vi "main.vi"() -> ()   [LabVIEW 2025]
panel:
  out "pNN50":dbl
  out "NN50":i16
  out "RMSSD":dbl
  out "stdRR":dbl format="%0.2f"
  out "meanRR":dbl format="%0.5f"
  out "deltaTime":dbl[](array[numeric])
  out "Time":dbl[](array[numeric])
  out "HRV(t)":cluster{dbl[], dbl[]}(graph)
  out "deltaPeakTimes":dbl[](array[numeric])
  out "peakTimes":dbl[](array[numeric])
  out "2Dsignal/peaks":dbl[][](array[numeric])
  out "ECG w peaks":dynamicdata(graph)
  out "# peaks":dbl
  out "Raw ECG":dbl[](graph)
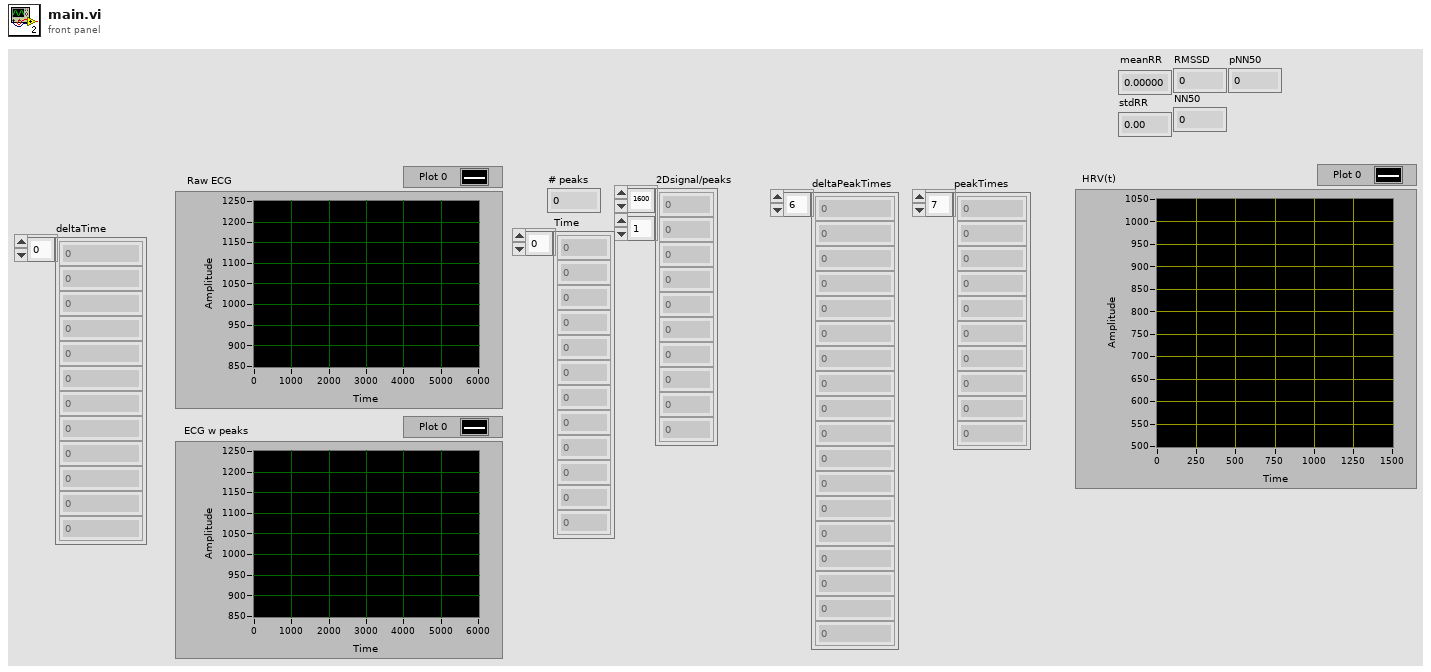
[diagram p1: front panel]
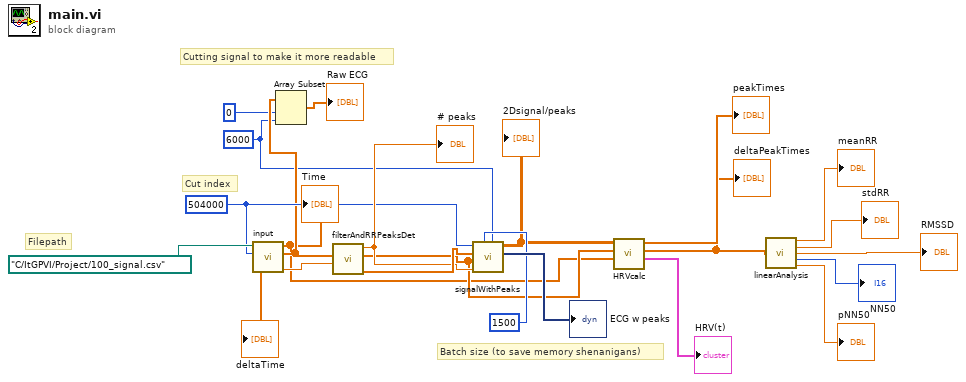
[diagram p0: block diagram]
diagram:
  w13 = 6000 ("length")
  w19 = 504000
  # "Batch size (to save memory shenanigans)"
  # "Cutting signal to make it more readable"
  # "Cut index"
  # "Filepath"
  n1 = call "input.vi"("cutIndex"=w19, "file path"=path "C:/ItGPVI/Project/100_signal.csv") -> ("fs"=w22:dbl, "ECG 1"=w16:dbl[], "Time"=w10:dbl[], "deltaTime"=→"deltaTime":dbl[])  [unwired: 4 in, 2 out]
  "Time" <- w10
  n2 = Array Subset(array=w16, index=0, length=w13) -> (→"Raw ECG":dbl[])
  n3 = call "filterAndRRPeaksDet.vi"("fs"=w22, "ECG1"=w16) -> ("Filtered ECG1"=w21:dbl[], "Locations"=w11:dbl[], "# peaks"=w20:dbl)  [unwired: 5 in, 2 out]
  "# peaks" <- w20
  n4 = call "signalWithPeaks.vi"("cutIndex"=w19, "filteredECG"=w21, "Locations"=w11, "# peaks"=w20, "batchSize"=1500, "lengthOfGraph"=w13) -> ("2Dsignal/peaks"=w12:dbl[][], "Waveform Graph"=→"ECG w peaks":dynamicdata)  [unwired: 3 in]
  "2Dsignal/peaks" <- w12
  n5 = call "HRVcalc.vi"("Time"=w10, "Locations"=w11, "2D"=w12) -> ("XY Graph"=→"HRV(t)":cluster{dbl[], dbl[]}, "deltaPeakTimes"=w6:dbl[], "peakTimes"=→"peakTimes":dbl[])  [unwired: 6 in]
  "deltaPeakTimes" <- w6
  n6 = call "linearAnalysis.vi"("deltaPeakTimes"=w6) -> ("meanRR"=→"meanRR":dbl, "stdRR"=→"stdRR":dbl, "RMSSD"=→"RMSSD":dbl, "NN50"=→"NN50":i16, "pNN50"=→"pNN50":dbl)  [unwired: 10 in]
